vi "MSEncoder SubVI ConfirmScanIndex.vi"(8 "error in (no error)":errorcluster, 10 "xml string":string, 11 "tdms file in":refnum<k34>) -> (0 "error out":errorcluster, 1 "UpdIndex":i32, 2 "ValueArray":dbl[](array[numeric]), 3 "tdms file out":refnum<k34>, 5 "Boolean":bool)   [LabVIEW 2018, in "MSEncoder.lvclass"]
uses:
  MSEncoder.lvclass
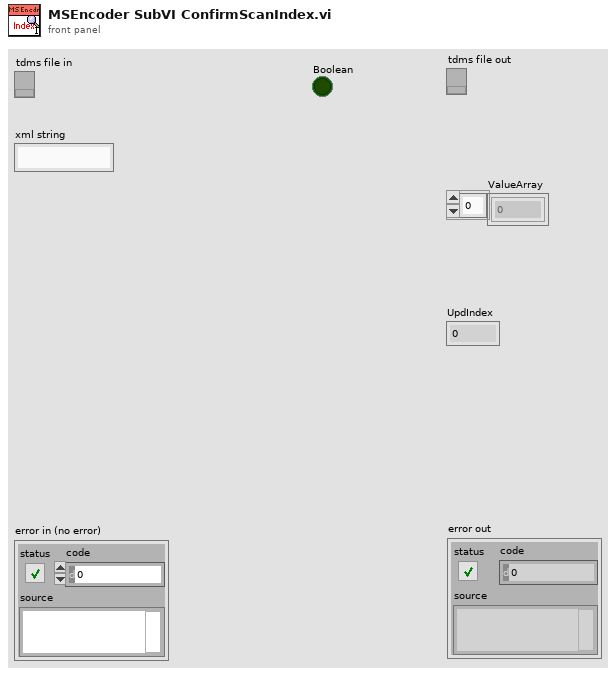
[diagram p1: front panel]
types:
  T1 = enum16{"open", "open or create", "create or replace", "create", "open (read-only)"}
  T2 = enum16{"open", "replace", "create", "open or create", "replace or create", "replace or create with confirmation"}
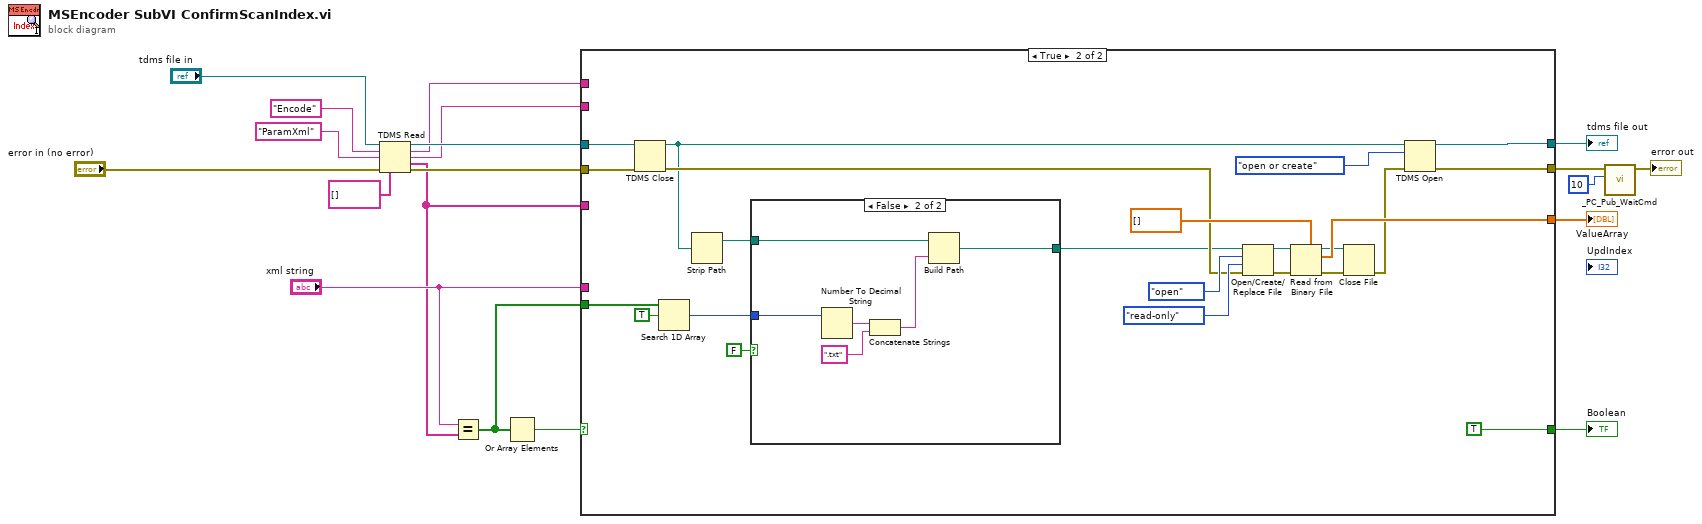
[diagram p0: block diagram]
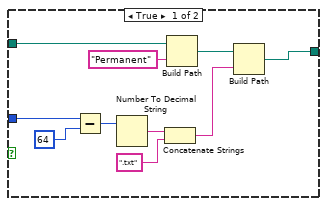
[diagram p3: hidden frame]
diagram:
  n1 = TDMS Read(0:"tdms file in", 5:"Encode" ("group name in (Untitled)"), 7:"ParamXml" ("channel name(s) in (Untitled)"), 11:"error in (no error)", 12:string[] []) -> (4:w13:refnum<k34>, 6:w10:string, 8:w9:string, 10:w5:string[], 15:w7:errorcluster)  [unwired: 3 in, 1 out]
  n2 = Equal?(x="xml string", y=w5) -> (x = y?=w8:bool[])
  n3 = Or Array Elements(Boolean array=w8) -> (logical OR=w1:bool)
  n4 = case shown="True" w1 {
    selector: w1 -> [w22 _]
    tunnel: "xml string" -> [_ _]
    tunnel: w13 -> [w21 w43]
    tunnel: [w21 w42] -> w18
    tunnel: w9 -> [_ _]
    tunnel: w10 -> [_ _]
    tunnel: w8 -> [_ w45]
    tunnel: [w22 TRUE] -> w17
    tunnel: [_ w41] -> w16
    tunnel: w7 -> [w20 w40]
    tunnel: [w20 w39] -> w2
    tunnel: w5 -> [_ _]
    frame False {
    }
    frame True {
      n5 = TDMS Close(8:w40, 11:w43) -> (0:w30:errorcluster, 3:w25:path)
      n6 = Search 1D Array(1D array=w45, element=TRUE) -> (index of element=w24:i32)  [unwired: 1 in]
      n7 = Strip Path(path=w25) -> (stripped path=w27:path)  [unwired: 1 out]
      n8 = case shown="False" FALSE {
        tunnel: w27 -> [w55 w59]
        tunnel: [w49 w57] -> w26
        tunnel: w24 -> [w48 w56]
        frame True {
          n9 = Subtract(x=w48, y=64) -> (x-y=w46:i32)
          n10 = Number To Decimal String(number=w46) -> (decimal integer string=w51:string)  [unwired: 1 in]
          n11 = Concatenate Strings(w51, ".txt" ("string")) -> (w50:string)
          n12 = Build Path(base path=w55, name or relative path="Permanent") -> (appended path=w53:path)
          n13 = Build Path(base path=w53, name or relative path=w50) -> (appended path=w49:path)
        }
        frame False {
          n14 = Number To Decimal String(number=w56) -> (decimal integer string=w61:string)  [unwired: 1 in]
          n15 = Concatenate Strings(w61, ".txt" ("string")) -> (w58:string)
          n16 = Build Path(base path=w59, name or relative path=w58) -> (appended path=w57:path)
        }
      }
      n17 = Open/Create/Replace File(file path (use dialog)=w26, error in=w30, operation (0:open)=T2."open", access (0:read/write)=enum16{"read/write", "read-only", "write-only"}."read-only") -> (refnum out=w35:refnum<file>, error out=w34:errorcluster)  [unwired: 2 in, 1 out]
      n18 = Read from Binary File(5:dbl[] [] ("WfmCode"), 8:w34, 11:w35) -> (0:w31:errorcluster, 2:w41:dbl[], 3:w32:refnum<file>)  [unwired: 3 in, 1 out]
      n19 = Close File(refnum=w32, error in=w31) -> (error out=w29:errorcluster)  [unwired: 1 out]
      n20 = TDMS Open(8:w29, 10:T1."open or create" ("operation (0:open)"), 11:w25) -> (0:w39:errorcluster, 3:w42:refnum<k34>)  [unwired: 4 in]
    }
  }
  "tdms file out" <- w18
  "Boolean" <- w17
  "ValueArray" <- w16
  n21 = call "_PC_Pub_WaitCmd.vi"("milliseconds to wait"=u32 10, "error in (no error)"=w2) -> ("error out"=→"error out":errorcluster)  [unwired: 9 in]
